vi "PPL_TRAJ_ABS_POSE_EST_EXECUTE.vi"(6 "Pass_Through_Time":dbl=-1.0 format="%33.4f", 8 "error in (no error)":errorcluster) -> (0 "error out":errorcluster)   [LabVIEW 2019]
uses:
  <vilib>/Rock Robotics/WPI/ThirdParty/JAS_Junk/TrajLib/Rotation2d_Minus.vi
  <vilib>/Rock Robotics/WPI/ThirdParty/JAS_Junk/TrajLib/Rotation2d_Plus.vi
  <vilib>/Rock Robotics/WPI/ThirdParty/JAS_Junk/TrajLib/Twist2d_Create.vi
  <vilib>/Rock Robotics/WPI/ThirdParty/JAS_Junk/TrajLib/Rotation2d_GetRadians.vi
  <vilib>/Rock Robotics/WPI/ThirdParty/JAS_Junk/TrajLib/VI/Util_GetTime_U32.vi
  <vilib>/Rock Robotics/WPI/ThirdParty/JAS_Junk/TrajLib/Rotation2d_UnaryMinus.vi
  <vilib>/Rock Robotics/WPI/ThirdParty/JAS_Junk/TrajLib/Rotation2d_RotateBy.vi
  <vilib>/Rock Robotics/WPI/ThirdParty/JAS_Junk/TrajLib/Rotation2d_CreateXY.vi
  <vilib>/Rock Robotics/WPI/ThirdParty/JAS_Junk/TrajLib/Util_CalcDist.vi
  Diff_Drive_System/PPL_DRIVE_GLOBALS.vi
  PPL_TRAJECTORY_GLOBALS.vi
  <vilib>/Rock Robotics/WPI/ThirdParty/JAS_Junk/TrajLib/Pose2d_Exp.vi
  <vilib>/Rock Robotics/WPI/ThirdParty/JAS_Junk/TrajLib/VI/Util_GetTime_U64.vi
  <vilib>/Rock Robotics/WPI/ThirdParty/JAS_Junk/TrajLib/Trajectory_Library.lvlib
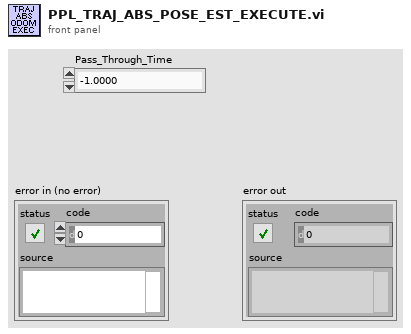
[diagram p1: front panel]
types:
  T1 = typedef "Trajectory_Library.lvlib/DIFF_DRIVE_KINEMATICS.ctl" = cluster{"TrackWidth_Meters":dbl}
  T2 = typedef "Trajectory_Library.lvlib/DIFF_DRIVE_ODOM2.ctl" = cluster{"M_POSE_Meters":T3, "M_GyroOffset":T5, "M_PrevAngle":T5, "M_PrevLeftDist_M":dbl, "M_PrevRightDist_M":dbl, "M_InitLeftDist_M":dbl, "M_InitRightDist_M":dbl}
  T3 = typedef "Trajectory_Library.lvlib/POSE2D.ctl" = cluster{"TRANSLATION":T4, "ROTATION":T5}
  T4 = typedef "Trajectory_Library.lvlib/TRANSLATION2D.ctl" = cluster{"X":dbl, "Y":dbl}
  T5 = typedef "Trajectory_Library.lvlib/ROTATION2D.ctl" = cluster{"VALUE":dbl, "COS":dbl, "SIN":dbl}
  T6 = typedef "Trajectory_Library.lvlib/DIFF_DRIVE_POSE_EST2_CONFIG.ctl" = cluster{"TrackWidth_Meters":dbl, "Odom X std dev M":dbl, "Odom Y std dev M":dbl, "Odom Heading std dev Rad":dbl, "Vision X std dev M":dbl, "Vision Y std dev M":dbl, "Vision Heading std dev Rad":dbl}
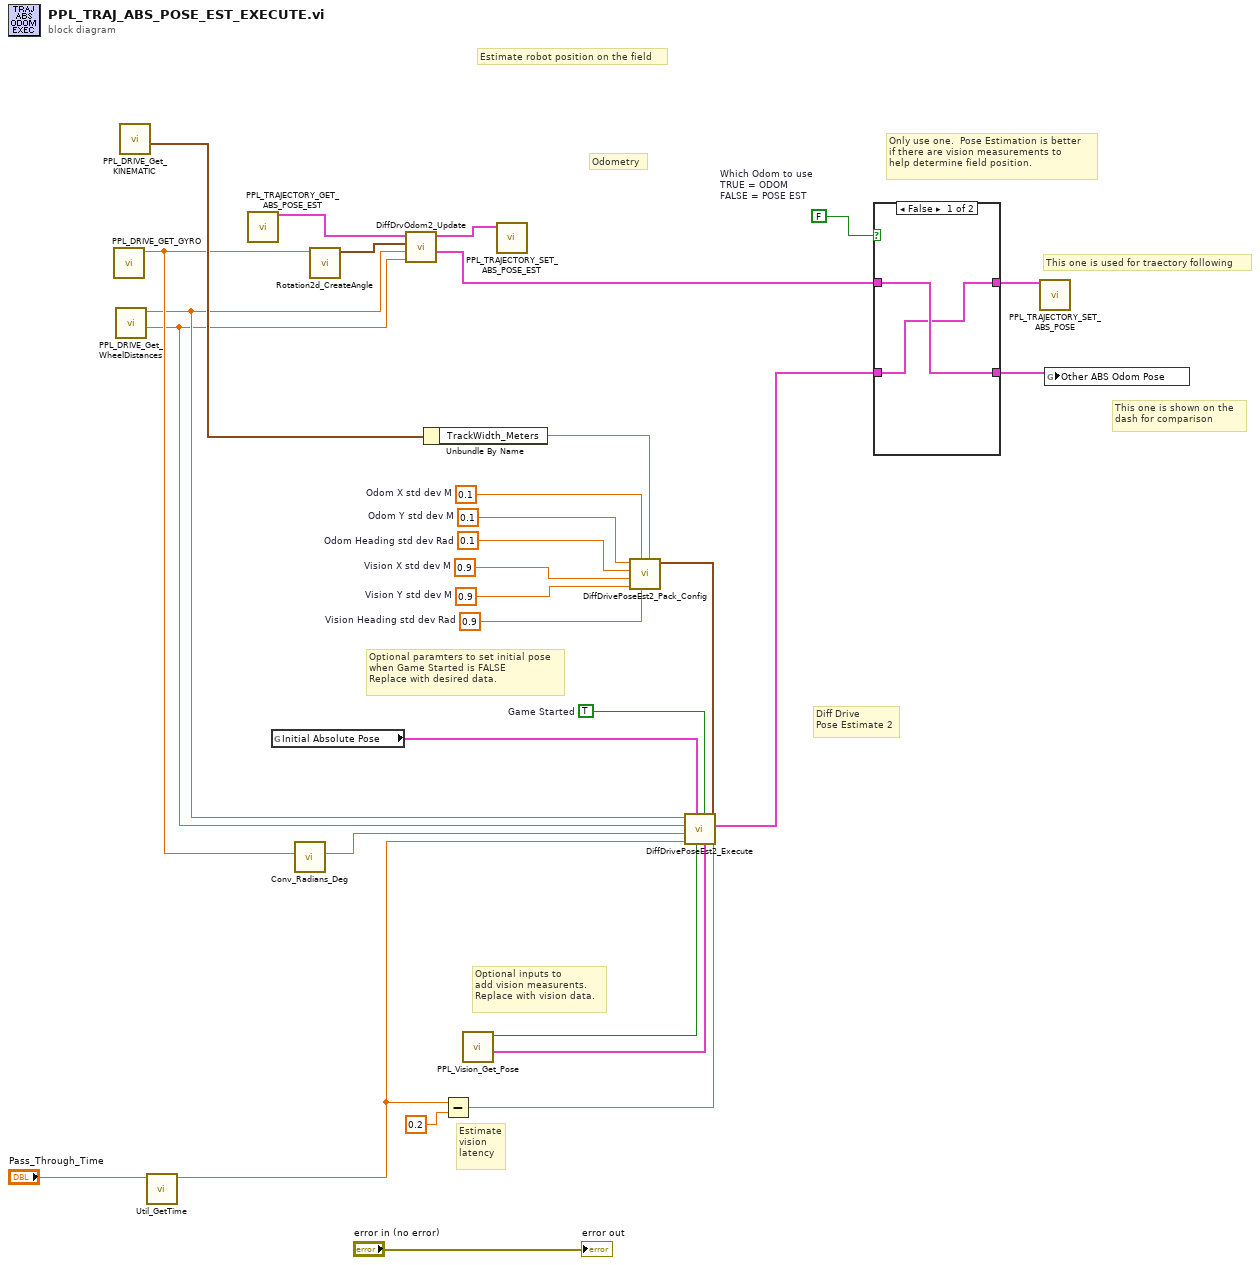
[diagram p0: block diagram]
diagram:
  w11 = FALSE  # Which Odom to use TRUE = ODOM FALSE = POSE EST
  w19 = TRUE  # Game Started
  w20 = 0.1  # Odom Y std dev M
  w21 = 0.1  # Odom Heading std dev Rad
  w22 = 0.9  # Vision X std dev M
  w23 = 0.9  # Vision Y std dev M
  w24 = 0.1  # Odom X std dev M
  w25 = 0.9  # Vision Heading std dev Rad
  # "Estimate\nvision \nlatency"
  # "This one is shown on the\ndash for comparison"
  # "This one is used for traectory following"
  # "Only use one.  Pose Estimation is better\nif there are vision measurements to\nhelp determine field position."
  # "Optional inputs to\nadd vision measurents.\nReplace with vision data."
  # "Optional paramters to set initial pose\nwhen Game Started is FALSE\nReplace with desired data."
  # "Diff Drive \nPose Estimate 2"
  # "Odometry"
  # "Estimate robot position on the field"
  n1 = call "PPL_DRIVE_GET_GYRO.vi"() -> ("Gyro Heading Radians"=w17:dbl)  [unwired: 11 in]
  n2 = call "PPL_DRIVE_Get_WheelDistances.vi"() -> ("Right Wheel Dist M"=w1:dbl, "Left Wheel Dist M"=w3:dbl)  [unwired: 10 in]
  n3 = call "PPL_DRIVE_Get_KINEMATIC.vi"() -> ("out DIFF_DRIVE_KINEMATICS"=w29:T1)  [unwired: 11 in]
  n4 = call <vilib>:"Util_GetTime.vi"("Pass_Through_Time"="Pass_Through_Time") -> ("FPGA_Time_Seconds"=w10:dbl)  [unwired: 8 in, 2 out]
  n5 = call "PPL_TRAJECTORY_GET_ABS_POSE_EST.vi"() -> ("Absolue Odometry"=w2:T2)  [unwired: 11 in]
  n6 = global read "PPL_TRAJECTORY_GLOBALS.vi" "Initial Absolute Pose"() -> (w18:T3)
  n7 = call <vilib>:"Conv_Radians_Deg.vi"("Radians"=w17) -> ("Degrees"=w16:dbl)  [unwired: 10 in]
  n8 = call <vilib>:"Rotation2d_CreateAngle.vi"("Angle"=w17) -> ("ROTATION"=w27:T5)  [unwired: 10 in]
  n9 = call <vilib>:"DiffDrvOdom2_Update.vi"("Right Distance M"=w1, "Left Distance M"=w3, "Gyro Reading"=w27, "In DIFF_DRIVE_ODOM"=w2) -> ("Pose Meters"=w15:T3, "Out DIFF_DRIVE_ODOM"=w26:T2)  [unwired: 6 in]
  n10 = Unbundle By Name(w29) -> ("TrackWidth_Meters"=w4:dbl)
  n11 = Subtract(x=w10, y=0.2) -> (x-y=w8:dbl)
  n12 = call "PPL_Vision_Get_Pose.vi"() -> ("Vison Pose"=w6:T3, "Have Vision Pose"=w7:bool)  [unwired: 10 in]
  n13 = call "PPL_TRAJECTORY_SET_ABS_POSE_EST.vi"("Absolue Odometry"=w26) -> ()  [unwired: 11 in]
  n14 = call <vilib>:"DiffDrivePoseEst2_Pack_Config.vi"("TrackWidth_Meters"=w4, "Vision Heading std dev Rad"=w25, "Odom X std dev M"=w24, "Vision Y std dev M"=w23, "Vision X std dev M"=w22, "Odom Heading std dev Rad"=w21, "Odom Y std dev M"=w20) -> ("DiffPoseEst2Config"=w5:T6)  [unwired: 4 in]
  n15 = call <vilib>:"DiffDrivePoseEst2_Execute.vi"("Vision TImeStamp_Seconds"=w8, "DiffPoseEst2Config"=w5, "visionRobotPose"=w6, "Game Started"=w19, "Add Vision Meas"=w7, "InitialPose"=w18, "Pass Through Time"=w10, "Gyro Degrees"=w16, "RightDistance_M"=w1, "LeftDistance_M"=w3) -> ("Estimated Pose"=w13:T3)  [unwired: 1 out]
  n16 = case shown="False" w11 {
    tunnel: w15 -> [w32 w34]
    tunnel: [w31 w34] -> w14
    tunnel: w13 -> [w31 w33]
    tunnel: [w32 w33] -> w12
    frame False {
    }
    frame True {
    }
  }
  n17 = call "PPL_TRAJECTORY_SET_ABS_POSE.vi"("Absolute Odometry Pose"=w14) -> ()  [unwired: 11 in]
  n18 = global write "PPL_TRAJECTORY_GLOBALS.vi" "Other ABS Odom Pose"(w12) -> ()
  "error out" <- "error in (no error)"
